vi "Display Intermed Text.vi"(0 "A":T1={"Array Num"=[1, 2, 3], "Decimal Index"=0, "stop"=FALSE}, 2 "B":T1={"Array Num"=[1, 2, 3], "Decimal Index"=0, "stop"=FALSE}, 3 "Digits":i32, 4 "Block Out":i32=-1) -> (5 "Results":string)   [LabVIEW 2025]
uses:
  Number.ctl
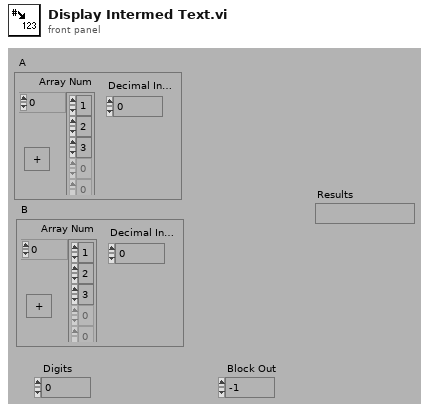
[diagram p1: front panel]
types:
  T1 = typedef "Number.ctl" = cluster{"Array Num":i8[], "Decimal Index":i32, "stop":bool}
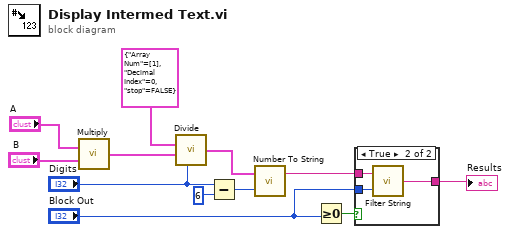
[diagram p0: block diagram]
diagram:
  n1 = call "Multiply.vi"("B"="B", "A"="A") -> ("Answer"=w1:T1)
  n2 = call "Divide.vi"("A"=T1 {"Array Num"=[1], "Decimal Index"=0, "stop"=FALSE}, "B"=w1, "digits"="Digits") -> ("A/B"=w6:T1)  [unwired: 2 in]
  n3 = Subtract(x="Digits", y=6 ("digit")) -> (x-y=w10:i32)
  n4 = call "Number To String.vi"("Digits"=w10, "Number"=w6) -> ("String"=w11:string)
  n5 = Greater Or Equal To 0?(x="Block Out") -> (x >= 0?=w7:bool)
  n6 = case shown="True" w7 {
    tunnel: w11 -> [w13 w16]
    tunnel: [w13 w15] -> w12
    tunnel: "Block Out" -> [_ w14]
    frame False {
    }
    frame True {
      n7 = call "Filter String.vi"("Index"=w14, "String In"=w16) -> ("String Out"=w15:string)
    }
  }
  "Results" <- w12
